vi "Export Custom Device Configuration.vi"(8 "error in (no error)":errorcluster, 10 "File Interface in":refnum<class "File Interface.lvclass">, 11 "ID":u64) -> (0 "error out":errorcluster, 3 "ID out":u64)   [LabVIEW 2015, in "ImportExport.lvlib"]
doc: "ExportCDConfig.vi saves a configuration file (.dat) that can be later loaded using ImportCDConfig.vi. This configuration file includes the values for the properties of each Section, Channel, or Waveform in your Custom Device. You can add this functionality as a Button, Runtime Menu, or as a property for one of your Channels."
uses:
  ImportExport.lvlib
  File Interface Class/File Interface.lvclass
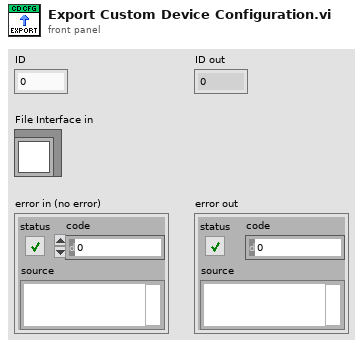
[diagram p1: front panel]
types:
  T1 = typedef "Advanced System Definition.lvlib/SysDef.Export.ctl" = cluster{"Version":string, "Tree":T2[]}
  T2 = typedef "Advanced System Definition.lvlib/TreeItem.ctl" = cluster{"Item Info":T3, "Parent Path":string[], "Properties":T8[]}
  T3 = typedef "Advanced System Definition.lvlib/TreeItem.Info.ctl" = cluster{"Name":string, "Description":string, "GUID":string, "Is Channel":bool, "Channel":T4, "Is Waveform":bool, "Waveform":T6}
  T4 = typedef "Custom Device API.lvlib/Custom Device Channel.ctl" = cluster{"Type":T5, "Units":string, "Default Value":dbl, "Faultable":bool, "Scalable":bool}
  T5 = typedef "Custom Device API.lvlib/Custom Device Channel Type.ctl" = enum16{"Input", "Output"}
  T6 = typedef "Custom Device API.lvlib/Custom Device Waveform.ctl" = cluster{"Data Type":T7, "Units":string}
  T7 = typedef "Custom Device API.lvlib/Custom Device Waveform DataType.ctl" = enum16{"Double", "Complex Double"}
  T8 = typedef "Advanced System Definition.lvlib/TreeItem.Property.ctl" = cluster{"Name":string, "Type":i32, "Value":variant}
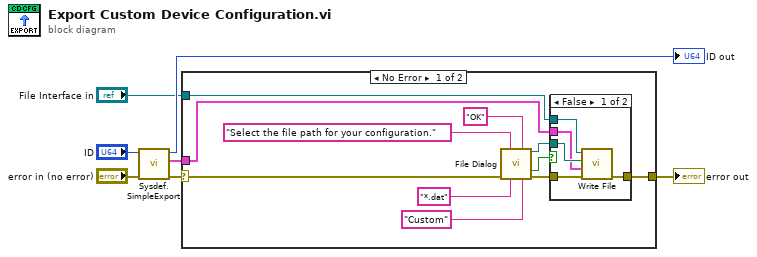
[diagram p0: block diagram]
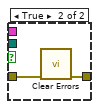
[diagram p2: hidden frame]
diagram:
  n1 = call "Sysdef.SimpleExport.vi"("error in (no error)"="error in (no error)", "ID"="ID") -> ("error out"=w7:errorcluster, "Export"=w6:T1, "ID out"=→"ID out":u64)  [unwired: 7 in]
  n2 = case shown="No Error" w7 {
    selector: w7 -> [w14 w26]
    tunnel: [w9 w26] -> w2
    tunnel: w6 -> [w10 _]
    tunnel: "File Interface in" -> [w8 _]
    frame No Error {
      n3 = call "File Dialog"("prompt"="Select the file path for your configuration.", "button label"="OK", "error in"=w14, "pattern (all files)"="*.dat", "pattern label"="Custom") -> ("selected path"=w11:path, "cancelled"=w13:bool, "error out"=w12:errorcluster)  [unwired: 7 in, 1 out]
      n4 = case shown="False" w13 {
        tunnel: [w19 w24] -> w9
        tunnel: w12 -> [w20 w25]
        tunnel: w11 -> [w22 _]
        tunnel: w10 -> [w21 _]
        tunnel: w8 -> [w23 _]
        frame False {
          n5 = call-dynamic "Write File.vi"("error in (no error)"=w20, "Data"=w21, "datalog path (use dialog)"=w22, "File Interface in"=w23) -> ("error out"=w19:errorcluster)  [unwired: 7 in]
        }
        frame True {
          n6 = call <vilib>:"Clear Errors.vi"("error in (no error)"=w25) -> ("error out"=w24:errorcluster)  [unwired: 5 in, 1 out]
        }
      }
    }
    frame Error {
    }
  }
  "error out" <- w2
